vi "CJ (SubVI).vi"(0 "jav pos":dbl[](array[numeric])=[0.2, 0.2, 0.5], 1 "Brake":bool, 4 "p_new":dbl[](array[numeric])=[2.0, 2.0, 0.0], 7 "error in":errorcluster, 8 "Go":bool, 9 "p_old":dbl[](array[numeric]), 10 "Eta":dbl[](array[numeric])=[0.0, 0.0, 0.0, 0.0, 0.0, 0.0], 13 "Theta des":dbl[](array[numeric])=[0.0, 0.0, 0.0, 0.0, 0.0, 0.0], 15 "time":dbl) -> (16 "Arrived":bool, 17 "p_ddot":dbl[](array[numeric]), 20 "javp":dbl[](array[numeric]), 25 "p_d":dbl[](array[numeric]), 26 "nu_d":dbl[](array[numeric]), 27 "error out":errorcluster)   [LabVIEW 2014]
uses:
  Library/Helping Routines/get_set_point_vec (SubVI).vi
  <vilib>/imath/engines/lvmath2/RunTimeEngine/IndexRead/NIMS V(S).vi
  <instcachedir>/0/NIMS V(S)_0488751826AF41519A22953C041130DC.lvgen/NIMS V(S)_0488751826AF41519A22953C041130DC_000.vi
  <vilib>/imathl/engines/lvmath/Functions/Error Handling/Create Error.vi
  <vilib>/imath/engines/lvmath2/RunTimeEngine/ArithmeticOperatorToken/NIMS_ArithmeticOperator_multmx(M,CV).vi
  <instcachedir>/0/NIMS_ArithmeticOperator_multmx(M,CV)_787B4652E60B4C52835A7FB23671E425.lvgen/NIMS_ArithmeticOperator_multmx(M,CV)_787B4652E60B4C52835A7FB23671E425_000.vi
  <vilib>/imath/engines/lvmath2/RunTimeEngine/NodeEndStatement/NIMS_NodeEndStatement_Get Vector.vi
  <instcachedir>/0/NIMS_NodeEndStatement_Get Vector_00D1625602D843AD9D7EC134A9EC13A2.lvgen/NIMS_NodeEndStatement_Get Vector_00D1625602D843AD9D7EC134A9EC13A2_001.vi
  <vilib>/imath/engines/lvmath2/RunTimeEngine/NodeEndStatement/NIMS_NodeEndStatement_Output.vi
  <instcachedir>/0/NIMS_NodeEndStatement_Output_53EC0D466D134D7ABD903AC30B43404B.lvgen/NIMS_NodeEndStatement_Output_53EC0D466D134D7ABD903AC30B43404B_005.vi
  <vilib>/imath/engines/lvmath2/RunTimeEngine/ErrorHandling/NIMS_Finalize Error.vi
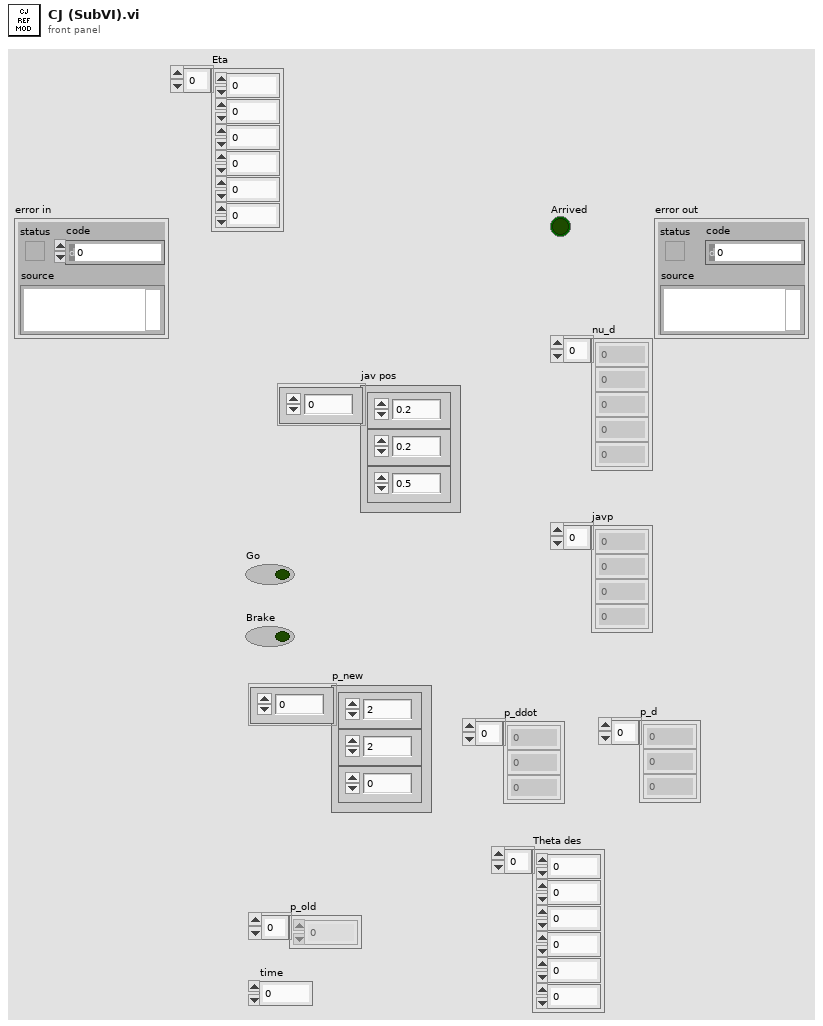
[diagram p1: front panel]
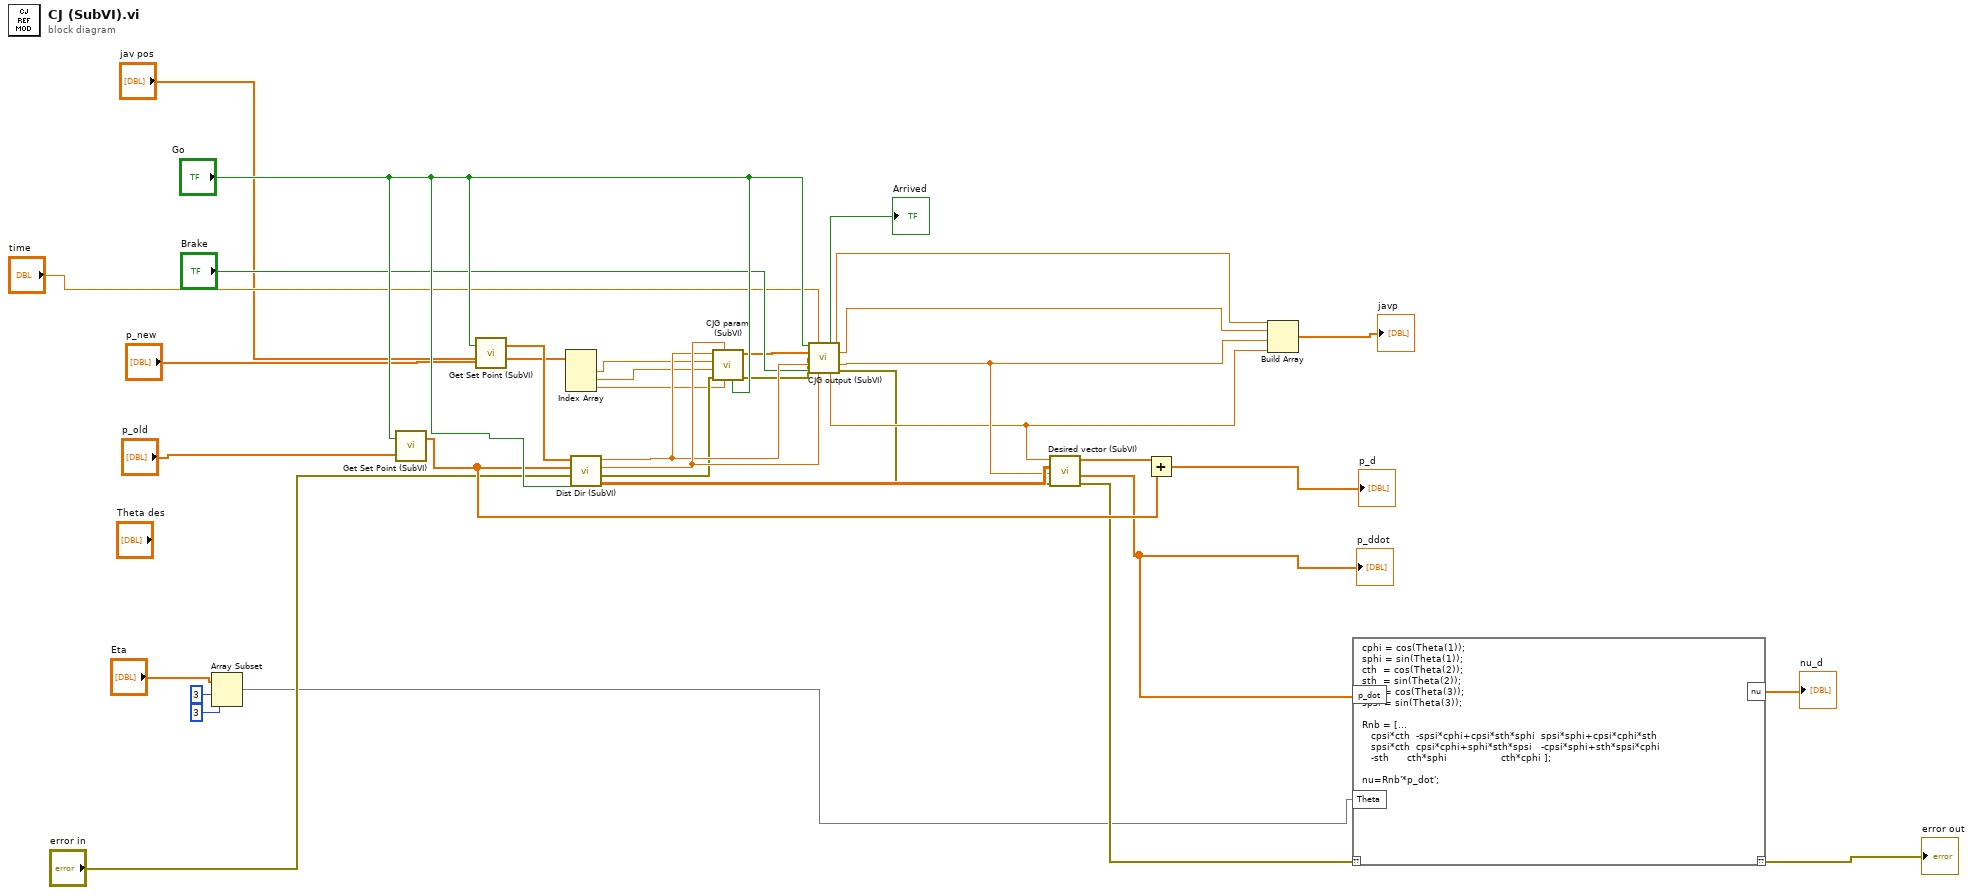
[diagram p0: block diagram]
diagram:
  n1 = Array Subset(array="Eta", index=3, length=3) -> (w1:dbl[])
  n2 = call-poly "Get Set Point (SubVI).vi"("Set point in"="p_old", "auto set  in"="Go") -> ("Set point"=w28:dbl[])  [unwired: 1 out]
  n3 = call-poly "Get Set Point (SubVI).vi"("Set point in"="p_new", "auto set  in"="Go") -> ("Set point"=w26:dbl[])  [unwired: 1 out]
  n4 = Index Array(array="jav pos") -> (element #1=w7:dbl, element #2=w6:dbl, element #3=w5:dbl)  [unwired: 3 in]
  n5 = call "Dist Dir (SubVI).vi"("Update"="Go", "error in"="error in", "p_0"=w28, "p_des"=w26) -> ("R_p"=w33:dbl[][], "error out"=w13:errorcluster, "p_m"=w32:dbl, "p0"=w31:dbl)  [unwired: 4 in]
  n6 = call "CJG param (SubVI).vi"("Boolean"="Go", "v_m"=w5, "p_m"=w32, "error in"=w13, "a_m"=w6, "j_m"=w7, "p_0"=w31) -> ("error out"=w12:errorcluster, "Array"=w23:dbl[])  [unwired: 3 in]
  n7 = call "CJG output (SubVI).vi"("Update"="Go", "time"="time", "parameters"=w23, "error in"=w12, "p_0"=w31, "Brake"="Brake", "p_m"=w32) -> ("Arrived"=→"Arrived":bool, "j"=w20:dbl, "a"=w19:dbl, "v"=w18:dbl, "p"=w17:dbl, "error out"=w11:errorcluster)  [unwired: 3 in]
  n8 = call "Desired vector (SubVI).vi"("error in"=w11, "v"=w18, "R_p"=w33, "p"=w17) -> ("error out"=w10:errorcluster, "p_ddot"=w22:dbl[], "p_d"=w29:dbl[])  [unwired: 1 in]
  "p_ddot" <- w22
  n9 = Add(x=w29, y=w28) -> (x+y=→"p_d":dbl[])
  n10 = Build Array(w20, w19, w18, w17) -> (→"javp":dbl[])
  n11 = mathscript code="cphi = cos(Theta(1));\nsphi = sin(Theta(1));\ncth  = cos(Theta(2));\nsth  = sin(Theta(2));\ncpsi = cos(Theta(3));\nspsi = sin(Theta(3));\n \nRnb = [...\n   cpsi*cth  -spsi*cphi+cpsi*sth*sphi  spsi*sphi+cpsi*cphi*sth\n   spsi*cth  cpsi*cphi+sphi*sth*spsi   -cpsi*sphi+sth*spsi*cphi\n   -sth      cth*sphi                  cth*cphi ];\n\nnu=Rnb'*p_dot';"("??"=w10, "Theta"=w1, "p_dot"=w22) -> ("??"=→"error out":errorcluster, "nu"=→"nu_d":dbl[])
